vi "S2C_M2p5942_Proc_LocalUpdate.vi"(8 "Error In":errorcluster, 10 "Data":string, 11 "Command":string) -> (0 "Error Out":errorcluster)   [LabVIEW 2024]
uses:
  S2C_M2p5942_Proc_Globals.vi
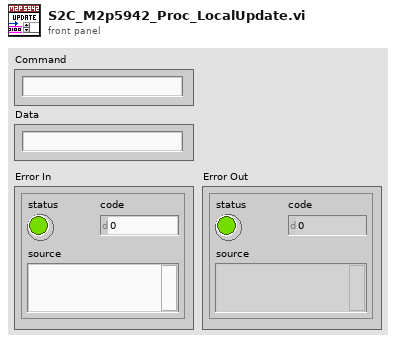
[diagram p1: front panel]
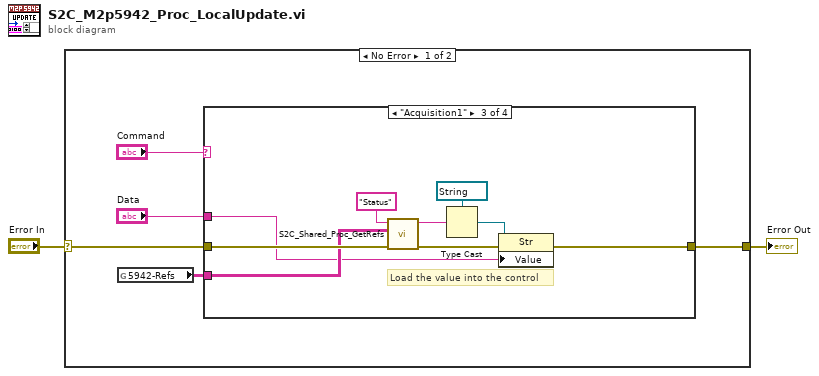
[diagram p0: block diagram]
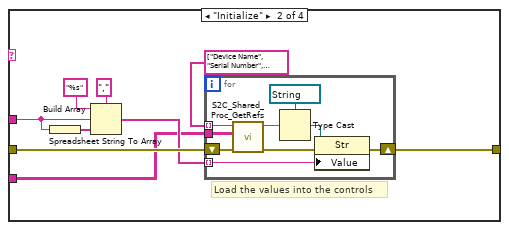
[diagram p3: hidden frame]
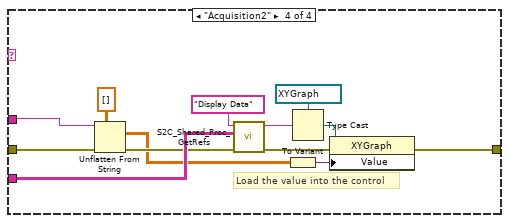
[diagram p4: hidden frame]
diagram:
  n1 = case shown="No Error" "Error In" {
    selector: "Error In" -> [w6 w49]
    tunnel: [w4 w49] -> w1
    frame No Error {
      n2 = global read "S2C_M2p5942_Proc_Globals.vi" "5942-Refs"() -> (w3:string[][])
      n3 = case shown="\"Acquisition1\"" "Command" {
        tunnel: w6 -> [w8 w13 w35 w41]
        tunnel: "Data" -> [_ w14 w27 w40]
        tunnel: [w8 w11 w34 w48] -> w4
        tunnel: w3 -> [_ w10 w33 w47]
        frame "Other", Default {
        }
        frame "Initialize" {
          # "Load the values into the controls"
          n4 = Build Array(w14) -> (w15:string[])
          n5 = Spreadsheet String To Array(delimiter (Tab)=",", format string="%s", spreadsheet string=w14, array type (2D Dbl)=w15) -> (array=w12:string[])
          n6 = for {
            tunnel: w12 -> [w20] mode=indexing
            tunnel: string[] ["Device Name", "Serial Number", "Memory (MB)"] -> [w21] mode=indexing
            shift-right: [w19] -> w11
            shift-left: w13 -> [w22]
            tunnel: w10 -> [w18]
            n7 = call "S2C_Shared_Proc_GetRefs.vi"("Error In"=w22, "Refs"=w18, "Label"=w21) -> ("Error Out"=w25:errorcluster, "Reference"=w23:string)  [unwired: 7 in]
            n8 = Type Cast(type=refnum<vi> refnum ("Enum"), x=w23) -> (*(type *) &x=w24:refnum<vi>)
            n9 = property class="Str"(reference=w24, error in=w25, "Value"=w20) -> (error out=w19:errorcluster)  [unwired: 1 out]
          }
        }
        frame "Acquisition1" {
          # "Load the value into the control"
          n10 = call "S2C_Shared_Proc_GetRefs.vi"("Error In"=w35, "Refs"=w33, "Label"="Status") -> ("Error Out"=w31:errorcluster, "Reference"=w29:string)  [unwired: 7 in]
          n11 = Type Cast(type=refnum<vi> refnum ("Enum"), x=w29) -> (*(type *) &x=w30:refnum<vi>)
          n12 = property class="Str"(reference=w30, error in=w31, "Value"=w27) -> (error out=w34:errorcluster)  [unwired: 1 out]
        }
        frame "Acquisition2" {
          # "Load the value into the control"
          n13 = Unflatten From String(type=sgl[][] [] ("appended array"), binary string=w40, error in (no error)=w41) -> (value=w36:sgl[][], error out=w38:errorcluster)  [unwired: 2 in, 1 out]
          n14 = call "S2C_Shared_Proc_GetRefs.vi"("Error In"=w38, "Refs"=w47, "Label"="Display Data") -> ("Error Out"=w45:errorcluster, "Reference"=w43:string)  [unwired: 7 in]
          n15 = To Variant(anything=w36) -> (Variant=w37:variant)
          n16 = Type Cast(type=refnum<vi> refnum ("Enum"), x=w43) -> (*(type *) &x=w44:refnum<vi>)
          n17 = property class="XYGraph"(reference=w44, error in=w45, "Value"=w37) -> (error out=w48:errorcluster)  [unwired: 1 out]
        }
      }
    }
    frame Error {
    }
  }
  "Error Out" <- w1
